vi "Load db Config Data to Controls.vi"(8 "error in (no error)":errorcluster, 9 "Control References Array":refnum<vi>[](array[refnum]), 10 "Data":string[](array[string])) -> (0 "error out":errorcluster)   [LabVIEW 2017]
panel:
  out "Array 2":variant[](array[variant])
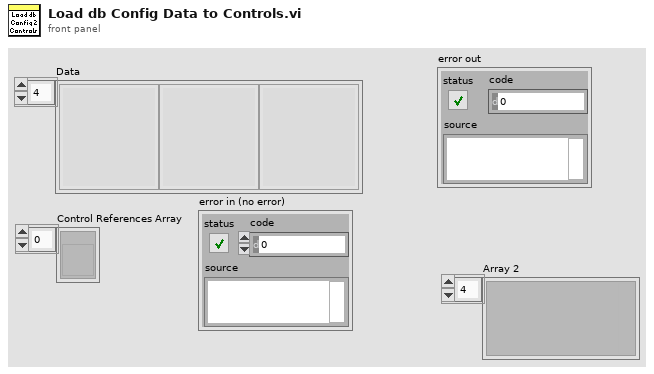
[diagram p1: front panel]
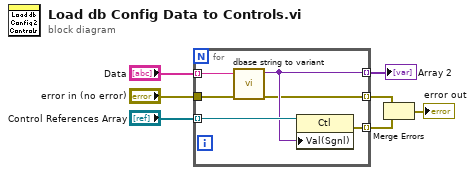
[diagram p0: block diagram]
diagram:
  n1 = for {
    tunnel: "Control References Array" -> [w13] mode=indexing
    tunnel: "Data" -> [w12] mode=indexing
    tunnel: [w11] -> w5 mode=indexing
    tunnel: "error in (no error)" -> [w10]
    tunnel: [w9] -> w3 mode=indexing
    tunnel: [w8] -> w2 mode=indexing
    n2 = call "dbase string to variant.vi"("error in (no error)"=w10, "String"=w12) -> ("error out"=w9:errorcluster, "Variant"=w11:variant)  [unwired: 8 in]
    n3 = property class="Ctl"(reference=w13, "Val(Sgnl)"=w11) -> (error out=w8:errorcluster)  [unwired: 1 in, 1 out]
  }
  "Array 2" <- w5
  n4 = Merge Errors(w3, w2) -> (→"error out":errorcluster)
